vi "Master, Record Step Name.vi"(7 "step name":string="Sequence Step General: Name", 8 "error in":errorcluster) -> (0 "error out":errorcluster)   [LabVIEW 2010]
doc: "This function displays the step name in the Master Record Results table."
panel:
  in  "dummy table":string[][](table) caption="Table 1"
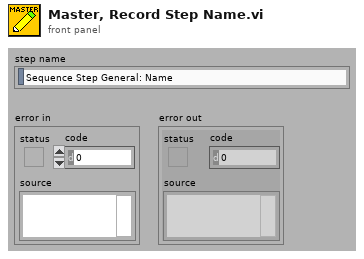
[diagram p1: front panel]
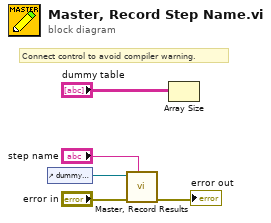
[diagram p0: block diagram]
diagram:
  # "Connect control to avoid compiler warning."
  n1 = control-ref of="dummy table"() -> (w5:refnum<vi>)
  n2 = call "Master, Record Results.vi"("step name"="step name", "error in"="error in", "Tbl Refnum"=w5) -> ("error out"=→"error out":errorcluster)  [unwired: 7 in, 1 out]
  n3 = Array Size(array="dummy table") -> ()  [unwired: 1 out]
